vi "Get Relay Control.vi"(5 "reset":bool caption="reset (optional)", 7 "state handshake":T2) -> (1 "stream.state n":T1, 2 "additive num samples":u16)   [LabVIEW 2015, in "niInstr Streaming v1 FPGA.lvlib"]
uses:
  <instrlib>/_niInstr/Streaming/v1/FPGA/niInstr Streaming v1 FPGA.lvlib
  <instrlib>/_niInstr/Streaming/v1/FPGA/Public/Stream Additive Count Register.ctl
  <instrlib>/_niInstr/Streaming/v1/Common/Stream State.ctl
  <instrlib>/_niInstr/Streaming/v1/FPGA/Public/Stream Additive Count Data.ctl
  <vilib>/rvi/Emulation/niFpgaSctlEmulationGetInTimedLoop.vi
  <vilib>/rvi/DataTransferAndStorage/Container/Common/niFpgaContainerExecOnDevCompGetState.vi
  <vilib>/rvi/Emulation/niFpgaEmulationIsFPGAContextNoSignature.vi
  <vilib>/rvi/DataTransferAndStorage/Container/Common/niFpgaContainerGetUniqueNameForEmu.vi
  <vilib>/rvi/eio/common/nirviEmuReportErrorAndStop.vi
  <vilib>/rvi/Emulation/niFpgaProcessEmulError.vi
  <vilib>/rvi/DataTransferAndStorage/Container/XNode/niFpgaContainer.xnode
  <vilib>/rvi/DataTransferAndStorage/Handshake/Emulation/niFpgaHandshakeEmulationRefIn.vi
  <instrlib>/_niInstr/Streaming/v1/Common/niInstr Streaming v1 Common.lvlib
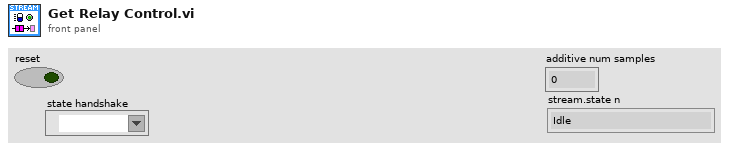
[diagram p1: front panel]
types:
  T1 = typedef "niInstr Streaming v1 Common.lvlib/Stream State.ctl" = enum8{"Idle", "Finite Transfer", "Continuous", "Done", "Error", "Not Ready", "Cancel"}
  T2 = typedef "niInstr Streaming v1 FPGA.lvlib/Stream Additive Count Register.ctl" = refnum<k21>
  T3 = typedef "niInstr Streaming v1 FPGA.lvlib/Stream Additive Count Data.ctl" = cluster{"stream.state":T1, "stream.additive num samples":u16}
  T4 = cluster{"stream.state":enum8{"Idle", "Finite Transfer", "Continuous", "Done", "Error", "Not Ready", "Cancel"}, "stream.additive num samples":u16}
  T5 = enum8{"Idle", "Finite Transfer", "Continuous", "Done", "Error", "Not Ready", "Cancel"}
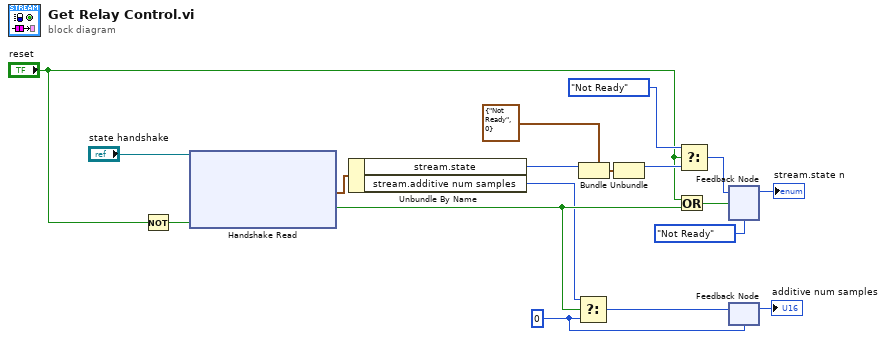
[diagram p0: block diagram]
diagram:
  w7 = u16 0 ("f")
  n1 = Not(x="reset") -> (.not. x?=w6:bool)
  n2 = xnode ("Handshake Read")("Ready for Output"=w6, "Handshake In"="state handshake") -> ("Data"=w17:T4, "Output Valid"=w15:bool)  [unwired: 1 out]
  n3 = Unbundle By Name(w17) -> ("stream.state"=w12:T5, "stream.additive num samples"=w9:u16)
  n4 = Select(t=w9, s=w15, f=w7) -> (s? t:f=w16:u16)
  n5 = Bundle(cluster=T3 {"stream.state"=enum."Not Ready", "stream.additive num samples"=0} ("Cluster"), "stream.state"=w12) -> (w11:T3)  [unwired: 1 in]
  n6 = Unbundle(w11) -> ("stream.state"=w3:T1)  [unwired: 1 out]
  n7 = Or(x="reset", y=w15) -> (x .or. y?=w5:bool)
  n8 = Select(t=Stream_State."Not Ready" ("stream.state 1"), s="reset", f=w3) -> (s? t:f=w2:T1)
  n9 = feedback-in #1(w2, w5) -> ()
  n10 = feedback #1(Stream_State."Not Ready" ("stream.state 1")) -> (→"stream.state n":T1)
  n11 = feedback #2(w7) -> (→"additive num samples":u16)
  n12 = feedback-in #2(w16) -> ()
